vi "from string.vi"(8 "error in":errorcluster, 9 "data":string, 10 "version":string, 11 "Tagbus PID Module configuration in":refnum<class "Tagbus PID Module configuration.lvclass">) -> (0 "error out":errorcluster, 3 "Tagbus PID Module configuration out":refnum<class "Tagbus PID Module configuration.lvclass">)   [LabVIEW 2014, in "Tagbus PID Module configuration.lvclass"]
doc: "Provides an interface for loading a module configuration from a file or other serialized data source. It is recommended that all children of this class store data in two sets--data required for its own initialization, and any data required for parent initialization--and that each implementation uses the <b>Call Parent Method</b> primitive to de-serialize parent information. As a result, it is expected that every module configuration class calls <b>component configuration.lvclass:From String.vi</b>."
uses:
  Tagbus PID Module configuration.lvclass
  Tagbus PID Module configuration.lvclass/Tagbus PID Module configuration.ctl
  <vilib>/NI/Tag Bus Module Framework/module configuration/TBM module configuration.lvclass
  <vilib>/NI/Configuration Framework/serializable configuration/NISE_CEF_serializable configuration.lvclass
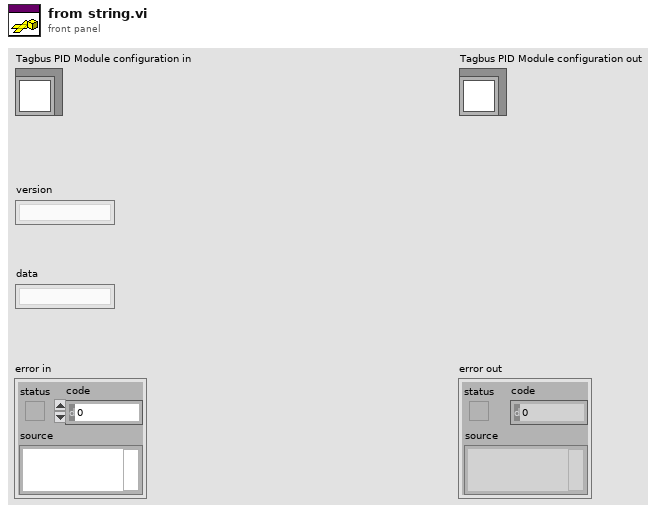
[diagram p1: front panel]
types:
  T1 = cluster{"Setpoint":refnum<class "TBM channel.lvclass">, "Process Variable":refnum<class "TBM channel.lvclass">, "Output":refnum<class "TBM channel.lvclass">, "PID gains":cluster{"proportional gain (Kc)":dbl, "integral time (Ti, min)":dbl, "derivative time (Td, min)":dbl}, "output range":cluster{"output high":dbl, "output low":dbl}, "ID":string}
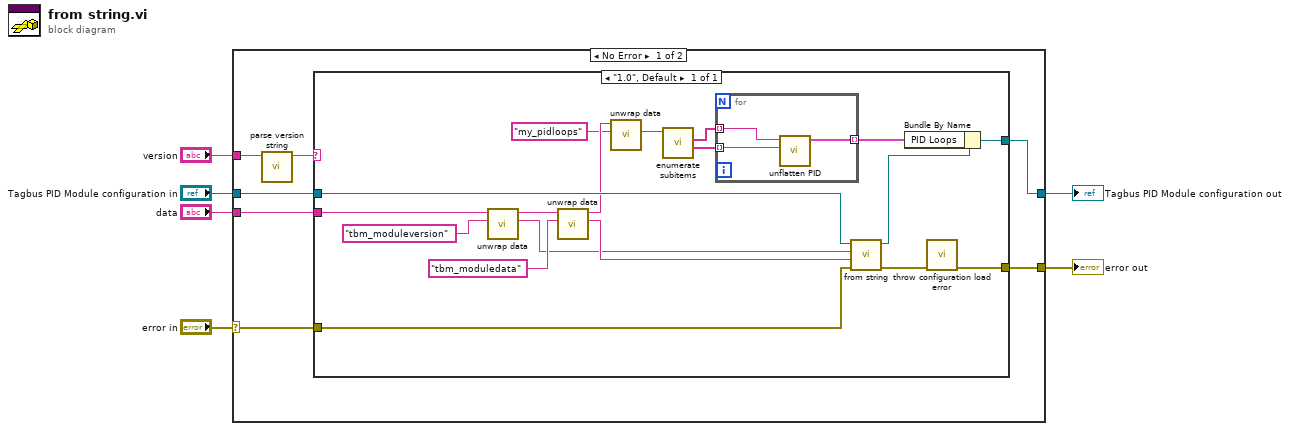
[diagram p0: block diagram]
diagram:
  n1 = case shown="No Error" "error in" {
    selector: "error in" -> [w7 w36]
    tunnel: "data" -> [w13 _]
    tunnel: "Tagbus PID Module configuration in" -> [w12 w35]
    tunnel: [w11 w35] -> w5
    tunnel: [w10 w36] -> w4
    tunnel: "version" -> [w9 _]
    frame No Error {
      n2 = call <vilib>:"parse version string.vi"("full version"=w9) -> ("major.minor version"=w8:string)  [unwired: 7 in, 3 out]
      n3 = case shown="\"1.0\", Default" w8 {
        tunnel: w13 -> [w28]
        tunnel: w7 -> [w27]
        tunnel: w12 -> [w31]
        tunnel: [w15] -> w11
        tunnel: [w30] -> w10
        frame "1.0", Default {
          n4 = call <vilib>:"unwrap data.vi"("identifier"="tbm_moduleversion" ("additional identifier"), "data to unwrap"=w28) -> ("unwrapped data"=w23:string, "remaining string"=w29:string)  [unwired: 8 in]
          n5 = call <vilib>:"unwrap data.vi"("identifier"="tbm_moduledata" ("additional identifier"), "data to unwrap"=w29) -> ("unwrapped data"=w25:string, "remaining string"=w22:string)  [unwired: 8 in]
          n6 = call <vilib>:"unwrap data.vi"("identifier"="my_pidloops" ("additional identifier"), "data to unwrap"=w22) -> ("unwrapped data"=w20:string)  [unwired: 8 in, 1 out]
          n7 = call <vilib>:"enumerate subitems.vi"("data to enumerate"=w20) -> ("associated data"=w18:string[], "discovered subitems"=w19:string[])  [unwired: 8 in, 1 out]
          n8 = for {
            tunnel: w19 -> [w34] mode=indexing
            tunnel: w18 -> [w32] mode=indexing
            tunnel: [w33] -> w14 mode=indexing
            n9 = call "unflatten PID.vi"("Identifier"=w32, "Data to Unwrap"=w34) -> ("Channels"=w33:T1)  [unwired: 9 in]
          }
          n10 = call-parent "from string.vi"("error in"=w27, "data"=w25, "version"=w23, "module configuration in"=w31) -> ("error out"=w17:errorcluster, "module configuration out"=w16:refnum<class "Tagbus PID Module configuration.lvclass">)  [unwired: 6 in]
          n11 = Bundle By Name(cluster=w16, "PID Loops"=w14) -> (w15:refnum<class "Tagbus PID Module configuration.lvclass">)
          n12 = call <vilib>:"throw configuration load error.vi"("error in"=w17) -> ("error out"=w30:errorcluster)  [unwired: 10 in]
        }
      }
    }
    frame Error {
    }
  }
  "error out" <- w4
  "Tagbus PID Module configuration out" <- w5
